vi "pump communication1.vi"() -> ()   [LabVIEW 2012]
uses:
  <vilib>/Instr/_visa.llb/VISA Configure Serial Port (Instr).vi
panel:
  in  "stop":bool
  out "return count":u32
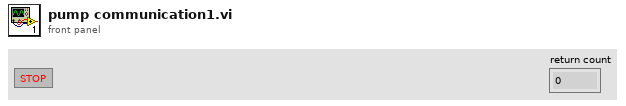
[diagram p1: front panel]
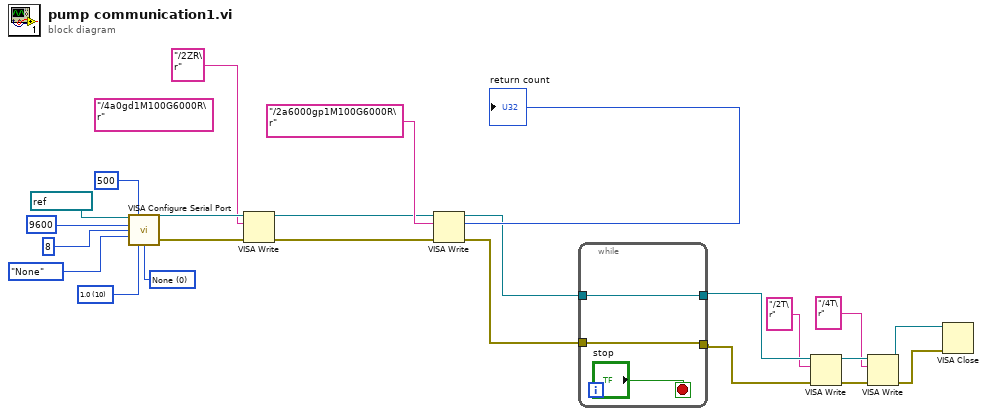
[diagram p0: block diagram]
diagram:
  (unwired) "/4a0gd1M100G6000R\r" ("write buffer")
  w17 = u16 0 items=["None", "XON/XOFF", "RTS/CTS", "XON/XOFF & RTS/CTS", "DTR/DSR", "XON/XOFF & DTR/DSR"] ("flow control (0:none)")
  w18 = u16 10 items=["1.0"=10, "1.5"=15, "2.0"=20] ("stop bits (10: 1 bit)")
  n1 = call-poly "VISA Configure Serial Port"("VISA resource name"=refnum<visa-resource-name> "COM4", "timeout (10sec)"=u32 500, "baud rate (9600)"=u32 9600, "data bits (8)"=u16 8, "parity (0:none)"=enum16{"None", "Odd", "Even", "Mark", "Space"}."None", "stop bits (10: 1 bit)"=w18, "flow control (0:none)"=w17) -> ("VISA resource name out"=w8:refnum<visa-resource-name>, "error out"=w7:errorcluster)  [unwired: 7 in]
  n2 = VISA Write(VISA resource name=w8, write buffer="/2ZR\r", error in (no error)=w7) -> (VISA resource name out=w10:refnum<visa-resource-name>, error out=w9:errorcluster)  [unwired: 1 out]
  n3 = VISA Write(VISA resource name=w10, write buffer="/2a6000gp1M100G6000R\r", error in (no error)=w9) -> (VISA resource name out=w14:refnum<visa-resource-name>, return count=→"return count":u32, error out=w15:errorcluster)
  n4 = while {
    tunnel: w15 -> [w26]
    tunnel: w14 -> [w25]
    tunnel: [w26] -> w13
    tunnel: [w25] -> w12
    stop <- "stop" stop-if-true
  }
  n5 = VISA Write(VISA resource name=w12, write buffer="/2T\r", error in (no error)=w13) -> (VISA resource name out=w3:refnum<visa-resource-name>, error out=w6:errorcluster)  [unwired: 1 out]
  n6 = VISA Write(VISA resource name=w3, write buffer="/4T\r", error in (no error)=w6) -> (VISA resource name out=w4:refnum<visa-resource-name>, error out=w5:errorcluster)  [unwired: 1 out]
  n7 = VISA Close(VISA resource name=w4, error in (no error)=w5) -> ()  [unwired: 1 out]
